vi "pre_modification.vi"(8 "error in (no error)":errorcluster, 11 "Instrument Command In":string) -> (0 "error out":errorcluster, 3 "Instrument Command Out":string)   [LabVIEW 2018]
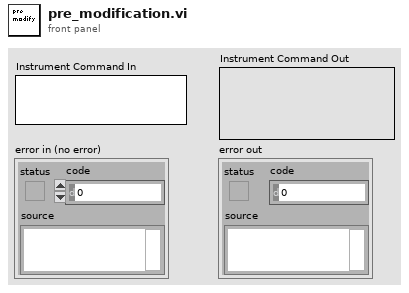
[diagram p1: front panel]
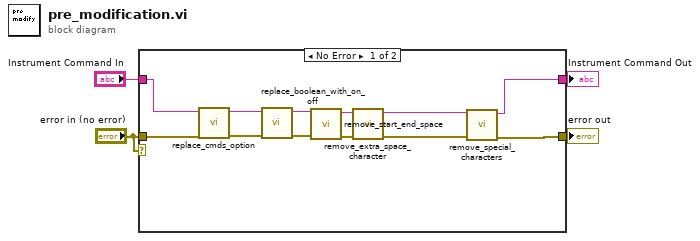
[diagram p0: block diagram]
diagram:
  n1 = case shown="No Error" "error in (no error)" {
    selector: "error in (no error)" -> [_ w18]
    tunnel: [w12 w18] -> w4
    tunnel: [w11 w17] -> w3
    tunnel: "error in (no error)" -> [w9 _]
    tunnel: "Instrument Command In" -> [w10 w17]
    frame No Error {
      n2 = call "replace_cmds_option.vi"("error in (no error)"=w9, "String In"=w10) -> ("error out"=w8:errorcluster, "String Out"=w7:string)  [unwired: 8 out]
      n3 = call "replace_boolean_with_on_off.vi"("error in (no error)"=w8, "String In"=w7) -> ("error out"=w13:errorcluster, "String Out"=w14:string)  [unwired: 8 out]
      n4 = call "remove_start_end_space.vi"("error in (no error)"=w13, "String"=w14) -> ("error out"=w16:errorcluster, "after substring"=w15:string)  [unwired: 8 out]
      n5 = call "remove_extra_space_character.vi"("error in (no error)"=w16, "Instrument Command In"=w15) -> ("error out"=w6:errorcluster, "Instrument Command Out"=w5:string)  [unwired: 8 out]
      n6 = call "remove_special_characters.vi"("error in (no error)"=w6, "Instrument Command In"=w5) -> ("error out"=w12:errorcluster, "Instrument Command Out"=w11:string)  [unwired: 8 out]
    }
    frame Error {
    }
  }
  "error out" <- w4
  "Instrument Command Out" <- w3
